vi "Get Stimulus Fit.vi"(8 "error in (no error)":errorcluster, 11 "Mean Fit in":refnum<class "Mean Fit.lvclass">) -> (0 "error out":errorcluster, 2 "Fit out":dbl[](array[numeric]), 3 "Mean Fit out":refnum<class "Mean Fit.lvclass">)   [LabVIEW 2013, in "Mean Fit.lvclass"]
uses:
  Mean Fit.lvclass
  Mean Fit.lvclass/Mean Fit.ctl
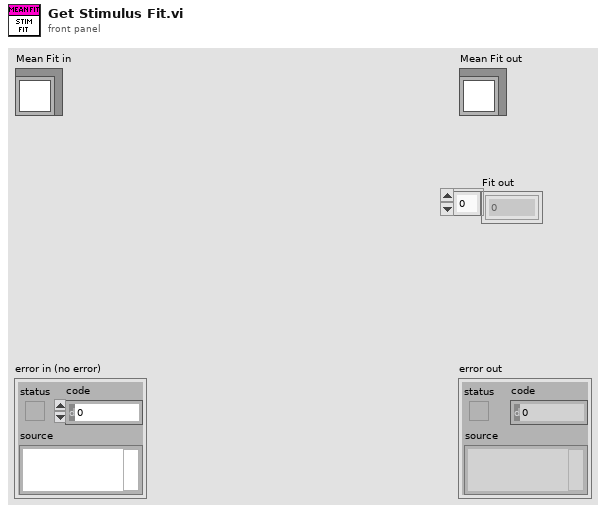
[diagram p1: front panel]
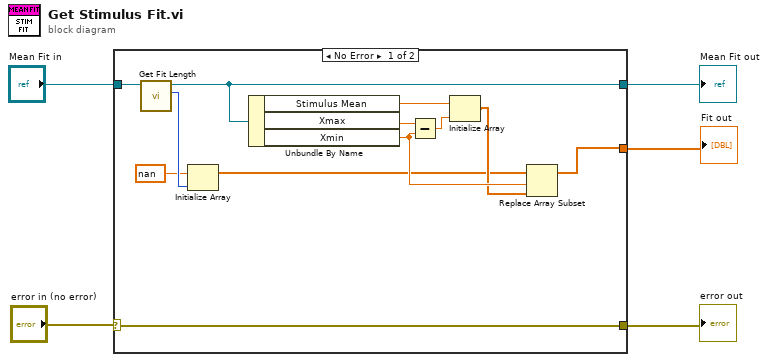
[diagram p0: block diagram]
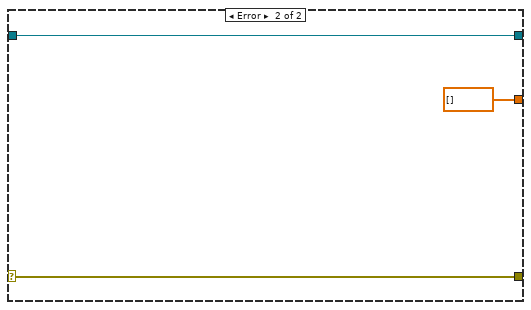
[diagram p2: hidden frame]
diagram:
  n1 = case shown="No Error" "error in (no error)" {
    selector: "error in (no error)" -> [w17 w20]
    tunnel: [w17 w20] -> w1
    tunnel: [w6 dbl[] [] ("Fit out")] -> w2
    tunnel: "Mean Fit in" -> [w16 w18]
    tunnel: [w13 w18] -> w3
    frame No Error {
      n2 = call-dynamic "Get Fit Length.vi"("Abstract Fit in"=w16) -> ("Length"=w15:i32, "Abstract Fit out"=w13:refnum<class "Mean Fit.lvclass">)  [unwired: 8 in, 1 out]
      n3 = Initialize Array(nan ("element"), w15) -> (w7:dbl[])
      n4 = Unbundle By Name(w13) -> ("Stimulus Mean"=w12:dbl, "Xmax"=w11:dbl, "Xmin"=w9:dbl)
      n5 = Subtract(x=w11, y=w9) -> (x-y=w10:dbl)
      n6 = Initialize Array(w12, w10) -> (w8:dbl[])
      n7 = Replace Array Subset(array=w7, new element=w8, index=w9) -> (w6:dbl[])
    }
    frame Error {
    }
  }
  "error out" <- w1
  "Mean Fit out" <- w3
  "Fit out" <- w2
